vi "VI server_Set Control Value from String Format.vi"(4 "Options":T1, 6 "Value.STR":string, 7 "Label":string, 8 "error in (no error)":errorcluster, 11 "VI Server Cluster":T2) -> (0 "error out":errorcluster, 1 "Control Reference (Generic)":refnum<vi>, 3 "VI Server Cluster.DUP":T2)   [LabVIEW 2020, in "VI Server Toolkit LV2013.lvlib"]
doc: "Sets control to value formatted as strings."
uses:
  VI Server Toolkit LV2013.lvlib
  VI Server_TypeDefs/VI Server_RefsCluster.ctl
  VI Server Libraries/VI Server Controls.llb/VI Server_GetSet Controls From String Format_Options.ctl
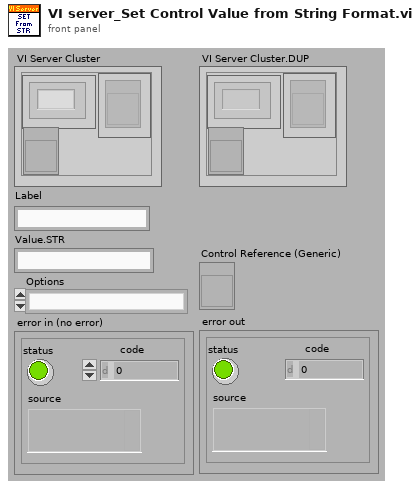
[diagram p1: front panel]
types:
  T1 = typedef "VI Server Toolkit LV2013.lvlib/VI Server_GetSet Controls From String Format_Options.ctl" = enum16{"", "If Ring Get Selection", "If Ring Set by Selection"}
  T2 = typedef "VI Server_RefsCluster.ctl" = cluster{"Labels":string[], "Refs":refnum<vi>[], "VI Ref":refnum<vi>}
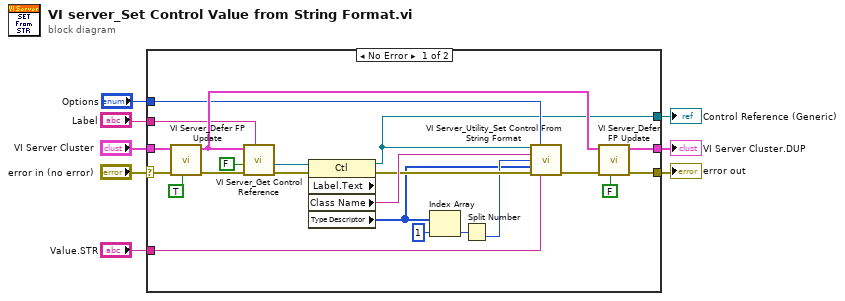
[diagram p0: block diagram]
diagram:
  n1 = case shown="No Error" "error in (no error)" {
    selector: "error in (no error)" -> [w26 w31]
    tunnel: "Label" -> [w11 _]
    tunnel: "Value.STR" -> [w27 _]
    tunnel: [w23 w31] -> w8
    tunnel: "VI Server Cluster" -> [w25 _]
    tunnel: [w20 _] -> w5
    tunnel: "Options" -> [w10 _]
    tunnel: [w9 _] -> w1
    frame No Error {
      n2 = call "VI Server_Defer FP Update.vi"("Defer Panel Updates? (F)"=TRUE ("Defer Panel Updates (F)"), "error in"=w26, "VI Server Cluster"=w25) -> ("error out"=w18:errorcluster, "VI Server Cluster.DUP"=w16:T2)  [unwired: 7 out]
      n3 = call "VI Server_Get Control Reference.vi"("Label"=w11, "error in"=w18, "Single Instance (T)"=FALSE, "VI Server Cluster"=w16) -> ("error out"=w17:errorcluster, "Control Reference (Generic)"=w12:refnum<vi>)  [unwired: 4 in, 2 out]
      n4 = property class="Ctl" props=["Label", "Text", "Class Name", "Type Descriptor"](reference=w12, error in=w17) -> (reference out=w9:refnum<vi>, error out=w29:errorcluster, "Class Name"=w30:string, "Type Descriptor"=w19:i16[])  [unwired: 1 out]
      n5 = Index Array(array=w19, index=1) -> (element=w13:i16)
      n6 = Split Number(x=w13) -> (lo(x)=w28:u8)  [unwired: 1 out]
      n7 = call "VI Server_Utility_Set Control From String Format.vi"("Control.Ref"=w9, "Options"=w10, "ClassName"=w30, "Control.Representation"=w28, "TypeDesc"=w19, "error in (no error)"=w29, "Value.STR"=w27) -> ("error out"=w22:errorcluster)  [unwired: 8 in]
      n8 = call "VI Server_Defer FP Update.vi"("Defer Panel Updates? (F)"=FALSE ("Defer Panel Updates (F)"), "error in"=w22, "VI Server Cluster"=w16) -> ("error out"=w23:errorcluster, "VI Server Cluster.DUP"=w20:T2)  [unwired: 7 out]
    }
    frame Error {
      n9 = call "VI Server_Empty VI Server Cluster.vi"() -> ()  [unwired: 7 in, 1 out]
    }
  }
  "error out" <- w8
  "VI Server Cluster.DUP" <- w5
  "Control Reference (Generic)" <- w1
